vi "BNO055 Example.vi"() -> ()   [LabVIEW 2017]
uses:
  <vilib>/MakerHub/LINX/Public/Utilities/Open Local.vi
  <vilib>/myRIO/Express VI/Onboard IO/DO/DO Express VI.xnode
  <vilib>/myRIO/Instrument Drivers/Onboard IO/DIO/vis/Write.vi
  <vilib>/myRIO/Instrument Drivers/Onboard IO/DIO/DIO.lvlib
  <vilib>/myRIO/Common/Instrument Driver Framework/myRIO v1.0/DIO/typedefs/DIO Channels Enum.ctl
  <vilib>/myRIO/Common/Instrument Driver Framework/myRIO v1.0/DIO/typedefs/DIO Channels List.ctl
  <vilib>/myRIO/Common/Instrument Driver Framework/Utilities/typedefs/Generic FPGA Reference.ctl
  <vilib>/myRIO/Common/Instrument Driver Framework/Utilities/typedefs/myRIO v1.0 Reference.ctl
  <vilib>/myRIO/Common/Instrument Driver Framework/Utilities/typedefs/Hardware Version Enum.ctl
  <vilib>/myRIO/Common/Instrument Driver Framework/Utilities/typedefs/myRIO Generic Hardware Reference.ctl
  <vilib>/myRIO/Instrument Drivers/Onboard IO/DIO/typedefs/DIO Reference.ctl
  <vilib>/myRIO/Instrument Drivers/Onboard IO/DIO/vis/myRIO DIO Open.xnode
  <vilib>/myRIO/Common/Instrument Driver Framework/Utilities/vis/Is FPGA Ref Available.vi
  <vilib>/myRIO/Common/Instrument Driver Framework/myRIO v1.0/DIO/vis/myRIO v1.1 Open DIO.vi
  <vilib>/userdefined/High Color/nirio_resource_hc.ctl
  IMU Control.ctl
panel:
  out "Gyr":cluster{"X":dbl, "Y":dbl, "Z":dbl}(graph)
  out "Mag":cluster{"X":dbl, "Y":dbl, "Z":dbl}(graph)
  out "Acc":cluster{"X":dbl, "Y":dbl, "Z":dbl}(graph)
  out "IMU":T1 {"Gyroscope"."Z" scale=-45.0..45.0; "Gyroscope"."Y" scale=-45.0..45.0; "Gyroscope"."X" scale=-45.0..45.0; "Magnetometer"."Z" scale=-2500.0..2500.0; "Magnetometer"."Y" scale=-2500.0..2500.0; "Magnetometer"."X" scale=-2500.0..2500.0; "Accelerometer"."Z" scale=-5.0..5.0; "Accelerometer"."Y" scale=-5.0..5.0; "Accelerometer"."X" scale=-5.0..5.0}
  in  "I2C Slave Address":u8=40 format="%x"
  in  "I2C Channel":u8=1
  out "Error Out":errorcluster
  out "Device Name":string
  out "ToF Loop Rate":u32
  in  "Wait (ms)":u32=10
  in  "Stop":bool
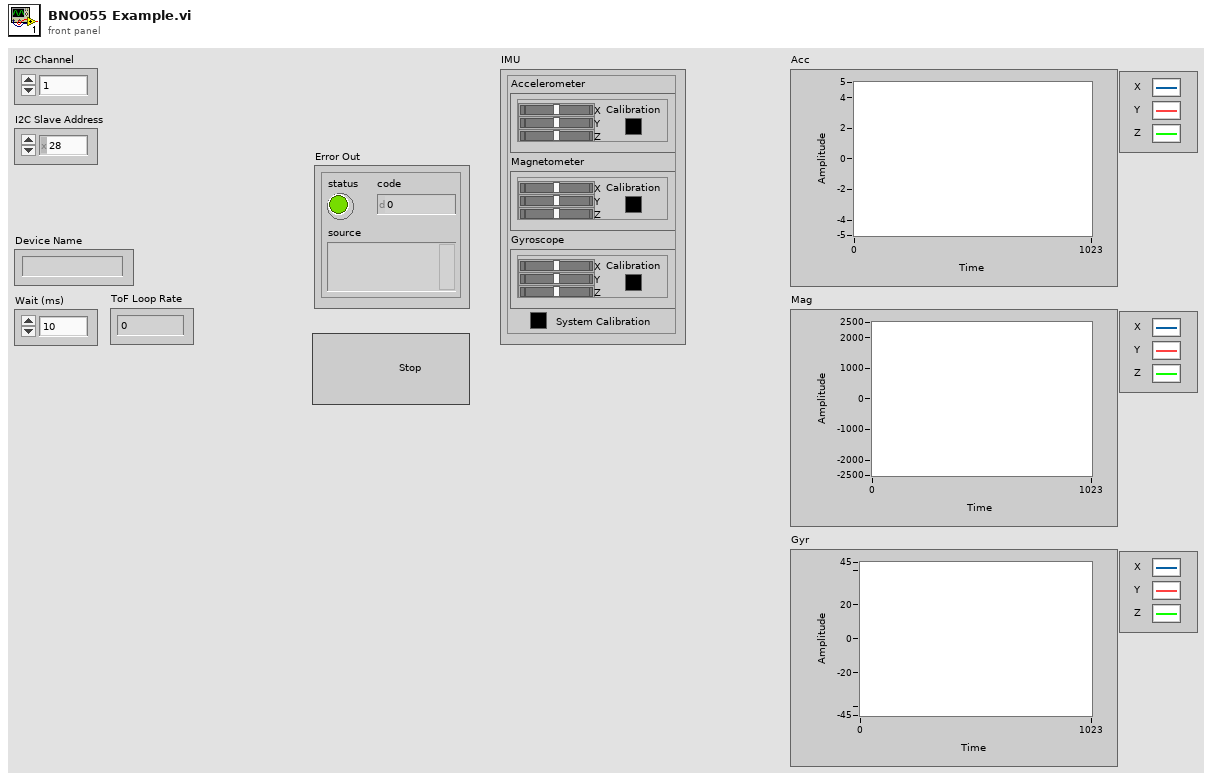
[diagram p1: front panel]
types:
  T1 = typedef "IMU Control.ctl" = cluster{"Accelerometer":cluster{"X":dbl, "Y":dbl, "Z":dbl, "Calibration":u32}, "Magnetometer":cluster{"X":dbl, "Y":dbl, "Z":dbl, "Calibration":u32}, "Gyroscope":cluster{"X":dbl, "Y":dbl, "Z":dbl, "Calibration":u32}, "System Calibration":u32}
  T2 = typedef "LMH-LINX.lvlib/LINX Ref.ctl" = cluster{"IO":T3, "Interface":T4, "LINX Device Config":T5}
  T3 = typedef "LMH-LINX.lvlib/Platform.ctl" = enum16{"Remote", "Local"}
  T4 = typedef "LMH-LINX.lvlib/Interface.ctl" = enum16{"Serial", "TCP"}
  T5 = typedef "LMH-LINX.lvlib/Device.lvlib/LINX Device Config.ctl" = cluster{"Interface":T4, "COM Port":refnum<visa-resource-name>, "TCP Configuration":T6, "Device Family":u8, "Device ID":u8, "Device Name":string, "TCP Ref":refnum<k5>, "Channels":T7}
  T6 = typedef "LMH-LINX.lvlib/Device.lvlib/TCP Config.ctl" = cluster{"IP Address":string, "Port":u16}
  T7 = typedef "LMH-LINX.lvlib/Channels.ctl" = cluster{"DI":u8[], "DO":u8[], "AI":u8[], "AO":u8[], "PWM":u8[], "QE":u8[], "UART":u8[], "I2C 2":u8[], "SPI":u8[], "CAN":u8[], "Servo":u8[], "AI Ref (V)":dbl, "AI Resolution (Bits)":u8, "AO Ref (V)":dbl, "AO Resolution (Bits)":u8}
  T8 = typedef "BNO055 Config Options.ctl" = cluster{"I2C":cluster{"Slave Address":u8, "Channel":u8}, "ADC":cluster{"Channel":u8, "Expected Range (Programmable Gain Amplifier)":u8, "Sampling Mode":u8, "Sampling Rate":u8, "Comparator Mode":u8, "Comparator Polarity":u8, "Latching Comparator":u8, "Comparator Queue & Disable":u8}}
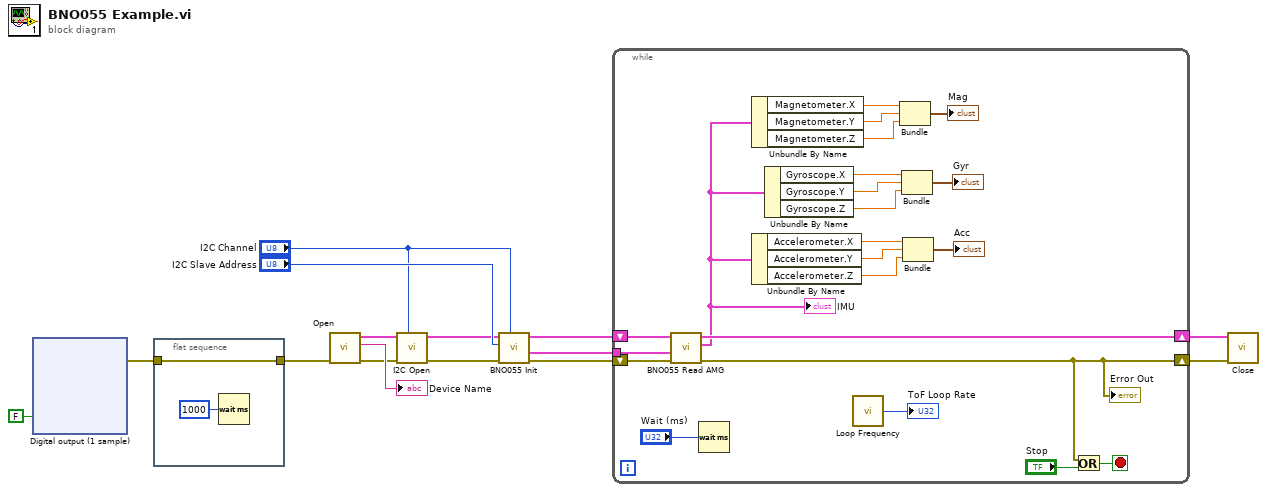
[diagram p0: block diagram]
diagram:
  n1 = xnode "Digital output (1 sample)"("Sensor Power (B/DIO7 (Pin 25))"=FALSE) -> ("error out"=w10:errorcluster)  [unwired: 1 in]
  n2 = flat-sequence {
    tunnel: w10 -> [w17]
    tunnel: [w17] -> w9
    frame #0 {
      n3 = Wait (ms)(milliseconds to wait=u32 1000) -> ()  [unwired: 1 out]
    }
  }
  n4 = call-poly <vilib>:"Open.vi"("Error In"=w9) -> ("Error Out"=w13:errorcluster, "Device Name"=→"Device Name":string, "LINX Resource"=w14:T2)  [unwired: 8 in]
  n5 = call <vilib>:"I2C Open.vi"("I2C Channel (0)"="I2C Channel", "Error In"=w13, "LINX Resource"=w14) -> ("Error Out"=w5:errorcluster, "LINX Resource"=w6:T2)  [unwired: 7 in]
  n6 = call "BNO055 Init.vi"("I2C Channel"="I2C Channel", "error in (no error)"=w5, "I2C Slave Address"="I2C Slave Address", "LINX Resource in"=w6) -> ("error out"=w4:errorcluster, "BNO055 Config Options 2"=w1:T8, "LINX Resource out"=w3:T2)  [unwired: 5 in]
  n7 = while {
    shift-right: [w35] -> w12
    shift-left: w3 -> [w38]
    shift-right: [w18] -> w11
    shift-left: w4 -> [w37]
    tunnel: w1 -> [w32]
    stop <- w34 stop-if-true
    n8 = call "BNO055 Read AMG.vi"("error in (no error)"=w37, "BNO055 Config Options"=w32, "LINX Resource in"=w38) -> ("error out"=w18:errorcluster, "IMU"=w19:T1, "LINX Resource"=w35:T2)  [unwired: 5 in, 1 out]
    "Error Out" <- w18
    "IMU" <- w19
    n9 = Wait (ms)(milliseconds to wait="Wait (ms)") -> ()  [unwired: 1 out]
    n10 = Unbundle By Name(w19) -> ("Magnetometer.X"=w23:dbl, "Magnetometer.Y"=w21:dbl, "Magnetometer.Z"=w22:dbl)
    n11 = Unbundle By Name(w19) -> ("Accelerometer.X"=w31:dbl, "Accelerometer.Y"=w29:dbl, "Accelerometer.Z"=w30:dbl)
    n12 = Unbundle By Name(w19) -> ("Gyroscope.X"=w27:dbl, "Gyroscope.Y"=w25:dbl, "Gyroscope.Z"=w26:dbl)
    n13 = call <vilib>:"Loop Frequency.vi"() -> ("Loop Rate (Hz)"=→"ToF Loop Rate":u32)
    n14 = Bundle("X"=w23, "Y"=w21, "Z"=w22) -> (→"Mag":cluster{"X":dbl, "Y":dbl, "Z":dbl})  [unwired: 1 in]
    n15 = Bundle("X"=w27, "Y"=w25, "Z"=w26) -> (→"Gyr":cluster{"X":dbl, "Y":dbl, "Z":dbl})  [unwired: 1 in]
    n16 = Bundle("X"=w31, "Y"=w29, "Z"=w30) -> (→"Acc":cluster{"X":dbl, "Y":dbl, "Z":dbl})  [unwired: 1 in]
    n17 = Or(x=w18, y="Stop") -> (x .or. y?=w34:bool)
  }
  n18 = call <vilib>:"Close.vi"("Error In"=w11, "LINX Resource"=w12) -> ()  [unwired: 9 in, 1 out]
